vi "VFH Speed Selection.vi"(6 "Histogram":dbl[](array[numeric]), 8 "Obstacle Clearance":dbl, 9 "Target Distance":dbl, 10 "Thresholds":T1, 11 "Max Speed":dbl) -> (3 "Speed":dbl)   [LabVIEW 2011]
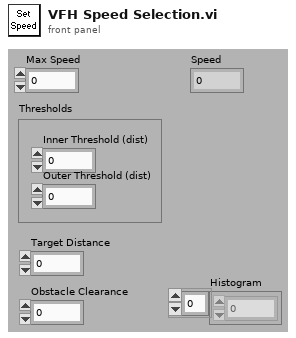
[diagram p1: front panel]
types:
  T1 = cluster{"Inner Threshold (dist)":dbl, "Outer Threshold (dist) ":dbl}
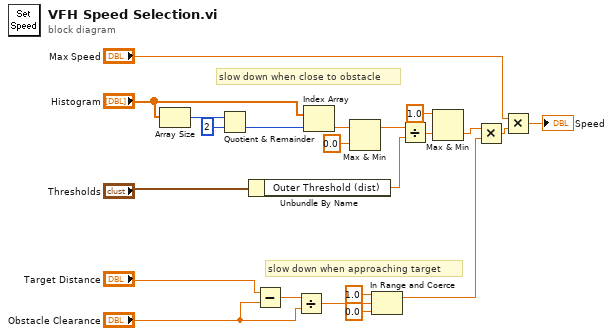
[diagram p0: block diagram]
diagram:
  # "slow down when close to obstacle"
  # "slow down when approaching target"
  n1 = Array Size(array="Histogram") -> (size(s)=w21:i32)
  n2 = Quotient & Remainder(x=w21, y=2) -> (floor(x/y)=w19:i32)  [unwired: 1 out]
  n3 = Unbundle By Name("Thresholds") -> ("Outer Threshold (dist)"=w13:dbl)
  n4 = Subtract(x="Target Distance", y="Obstacle Clearance") -> (x-y=w6:dbl)
  n5 = Divide(x=w6, y="Obstacle Clearance") -> (x/y=w5:dbl)
  n6 = Index Array(array="Histogram", index=w19) -> (element=w18:dbl)
  n7 = Max & Min(x=w18, y=0.0) -> (max(x,y)=w16:dbl)  [unwired: 1 out]
  n8 = In Range and Coerce(upper limit=1.0, x=w5, lower limit=0.0) -> (coerced(x)=w2:dbl)  [unwired: 1 out]
  n9 = Divide(x=w16, y=w13) -> (x/y=w12:dbl)
  n10 = Max & Min(x=1.0, y=w12) -> (min(x,y)=w10:dbl)  [unwired: 1 out]
  n11 = Multiply(x=w10, y=w2) -> (x*y=w3:dbl)
  n12 = Multiply(x="Max Speed", y=w3) -> (x*y=→"Speed":dbl)
